vi "Clear Scan Time Out1_2.vi"(7 "ESP32 ref":refnum<visa-resource-name>="COM4", 8 "error in (no error)":errorcluster, 11 "VISA Refnum in":refnum<visa-resource-name>) -> (0 "error out":errorcluster, 1 "error?":bool, 2 "Time out count":i32, 3 "VISA Refnum out":refnum<visa-resource-name>, 5 "ESP32 ref out":refnum<visa-resource-name>)   [LabVIEW 2023]
uses:
  <vilib>/Utility/error.llb/DialogType.ctl
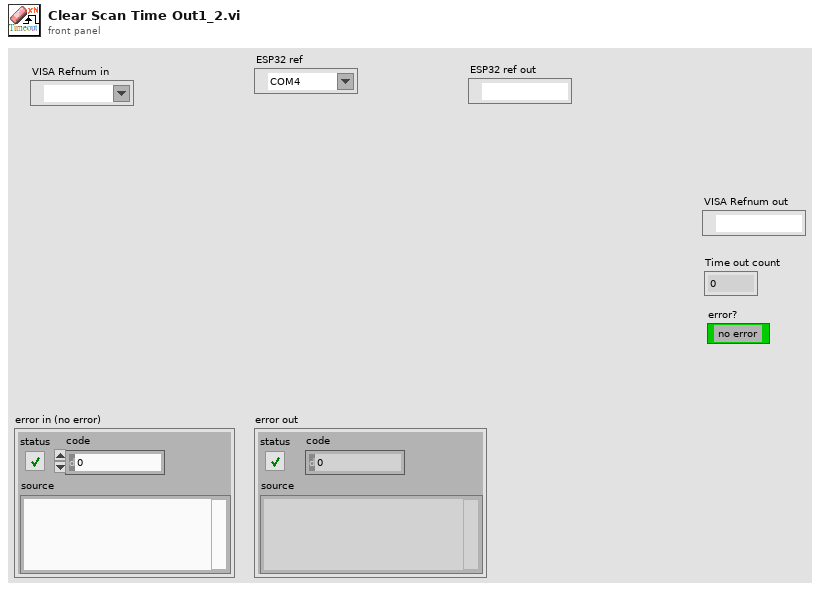
[diagram p1: front panel]
types:
  T1 = typedef "DialogType.ctl" = u16
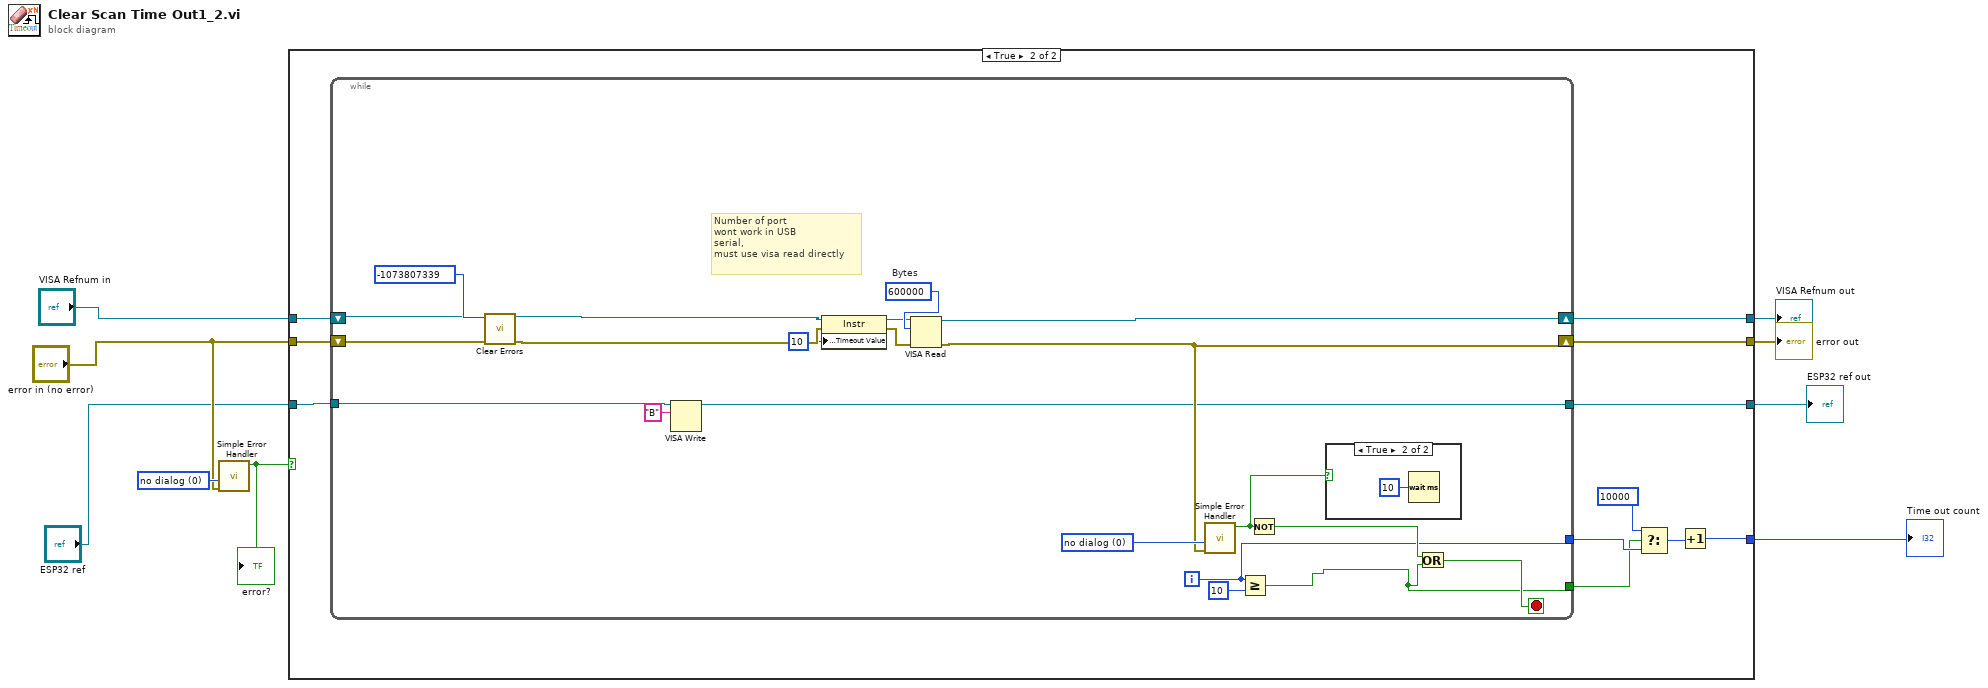
[diagram p0: block diagram]
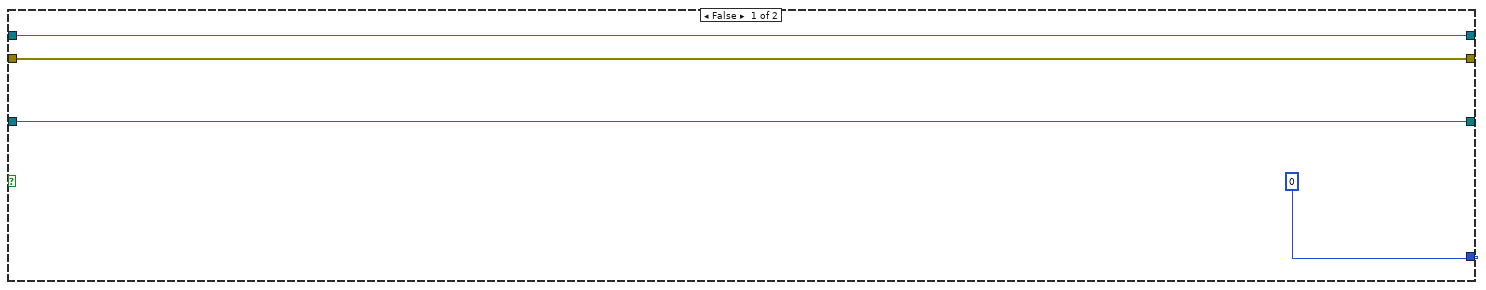
[diagram p2: hidden frame]
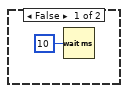
[diagram p3: hidden frame]
diagram:
  w6 = T1 0 items=["no dialog", "OK message", "continue or stop message", "OK message + warnings", "continue/stop + warnings"] ("type of dialog (OK msg:1)")
  n1 = call <vilib>:"Simple Error Handler.vi"("type of dialog (OK msg:1)"=w6, "error in (no error)"="error in (no error)") -> ("error?"=w4:bool)  [unwired: 3 in, 4 out]
  "error?" <- w4
  n2 = case shown="True" w4 {
    tunnel: [w13 w24] -> w9
    tunnel: "error in (no error)" -> [w12 w23]
    tunnel: "VISA Refnum in" -> [w13 w22]
    tunnel: [w12 w21] -> w7
    tunnel: [0 w20] -> w3
    tunnel: "ESP32 ref" -> [w10 w15]
    tunnel: [w10 w14] -> w1
    frame False {
    }
    frame True {
      n3 = while {
        shift-right: [w39] -> w21
        shift-left: w23 -> [w42]
        shift-right: [w44] -> w24
        shift-left: w22 -> [w28]
        tunnel: [w35] -> w18
        tunnel: [w25] -> w17
        tunnel: w15 -> [w27]
        tunnel: [w26] -> w14
        i -> [w35]
        stop <- w36 stop-if-true
        w32 = u32 600000  # Bytes
        w40 = T1 0 items=["no dialog", "OK message", "continue or stop message", "OK message + warnings", "continue/stop + warnings"] ("type of dialog (OK msg:1)")
        # "Number of port\nwont work in USB \nserial,\nmust use visa read directly"
        n4 = call <vilib>:"Clear Errors.vi"("error in (no error)"=w42, "specific error code to clear (0: all)"=-1073807339 ("code out")) -> ("error out"=w41:errorcluster)  [unwired: 4 in, 1 out]
        n5 = VISA Write(VISA resource name=w27, write buffer="B") -> (VISA resource name out=w26:refnum<visa-resource-name>)  [unwired: 1 in, 2 out]
        n6 = property class="Instr"(reference=w28, error in=w41, "General Settings:Timeout Value"=u32 10) -> (reference out=w31:refnum<visa-resource-name>, error out=w30:errorcluster)
        n7 = VISA Read(VISA resource name=w31, byte count=w32, error in (no error)=w30) -> (VISA resource name out=w44:refnum<visa-resource-name>, error out=w39:errorcluster)  [unwired: 2 out]
        n8 = call <vilib>:"Simple Error Handler.vi"("type of dialog (OK msg:1)"=w40, "error in (no error)"=w39) -> ("error?"=w34:bool)  [unwired: 3 in, 4 out]
        n9 = Greater Or Equal?(x=w35, y=10) -> (x >= y?=w25:bool)
        n10 = Not(x=w34) -> (.not. x?=w37:bool)
        n11 = case shown="True" w34 {
          frame False {
            n12 = Wait (ms)(milliseconds to wait=u32 10) -> ()  [unwired: 1 out]
          }
          frame True {
            n13 = Wait (ms)(milliseconds to wait=u32 10) -> ()  [unwired: 1 out]
          }
        }
        n14 = Or(x=w37, y=w25) -> (x .or. y?=w36:bool)
      }
      n15 = Select(t=10000, s=w17, f=w18) -> (s? t:f=w19:i32)
      n16 = Increment(x=w19) -> (x+1=w20:i32)
    }
  }
  "error out" <- w7
  "VISA Refnum out" <- w9
  "Time out count" <- w3
  "ESP32 ref out" <- w1
